vi "Print File.vi"(8 "error in (no error)":errorcluster, 9 "#Copies (1)":i16=1, 10 "Printer Name (default)":string, 11 "File Path":path) -> (0 "error out":errorcluster, 3 "ERROR":bool)   [LabVIEW 2017]
doc: "Prints the document located at the <b>File Path</b> location.\n\nThis VI uses the Windows PrintDocument .NET by creating an instance of the PrintDocument class, setting properties such as the DocumentName and PrinterSettings (PrinterName, number of Copies), and calling the Print method to start the printing process."
uses:
  user32.dll
  shell32.dll
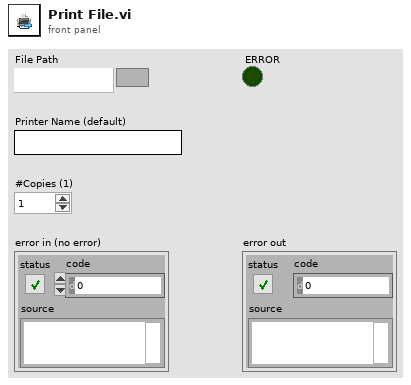
[diagram p1: front panel]
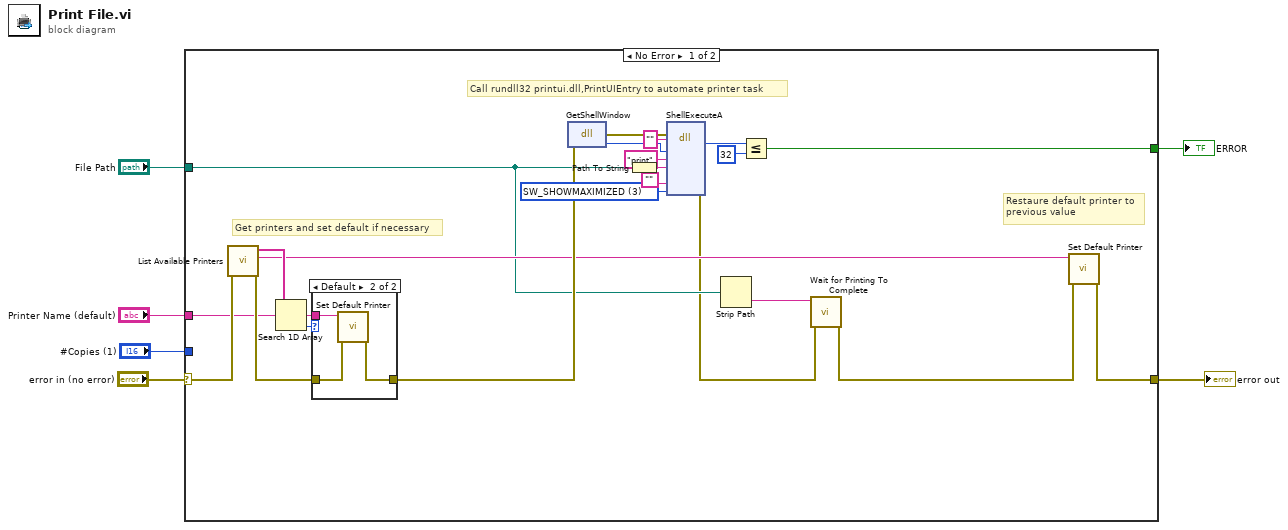
[diagram p0: block diagram]
diagram:
  n1 = case shown="No Error" "error in (no error)" {
    selector: "error in (no error)" -> [w26 w33]
    tunnel: "Printer Name (default)" -> [w12 _]
    tunnel: "File Path" -> [w10 _]
    tunnel: [w19 w33] -> w3
    tunnel: "#Copies (1)" -> [_ _]
    tunnel: [w13 _] -> w1
    frame No Error {
      w16 = u16 3 items=["SW_HIDE", "SW_NORMAL", "SW_SHOWMINIMIZED", "SW_SHOWMAXIMIZED", "SW_SHOWNOACTIVATE", "SW_SHOW", "SW_MINIMIZE", "SW_SHOWMINNOACTIVE", "SW_SHOWNA", "SW_RESTORE", "SW_SHOWDEFAULT", "SW_FORCEMINIMIZE"] ("Flag")
      # "Call rundll32 printui.dll,PrintUIEntry to automate printer task"
      # "Get printers and set default if necessary"
      # "Restaure default printer to\nprevious value"
      n2 = call "List Available Printers.vi"("error in (no error)"=w26) -> ("error out"=w27:errorcluster, "Default Printer"=w11:string, "Available Printers"=w28:string[])  [unwired: 8 in]
      n3 = Search 1D Array(1D array=w28, element=w12) -> (index of element=w14:i32)  [unwired: 1 in]
      n4 = case shown="Default" w14 {
        tunnel: w12 -> [_ w30]
        tunnel: w27 -> [w29 w32]
        tunnel: [w29 w31] -> w20
        frame -1 {
        }
        frame Default {
          n5 = call "Set Default Printer.vi"("error in (no error)"=w32, "Printer Name"=w30) -> ("error out"=w31:errorcluster)  [unwired: 9 in]
        }
      }
      n6 = dll-call lib="user32.dll" fn="GetShellWindow" label="user32.dll -> GetShellWindow"(error in=w20) -> (error out=w25:errorcluster, w24:u32)  [unwired: 2 in, 1 out]
      n7 = Path To String(path=w10) -> (string=w22:string)
      n8 = dll-call lib="shell32.dll" fn="ShellExecuteA" label="shell32.dll ->ShellExecuteA"(error in=w25, "hwnd"=w24, "lpOperation"="print", "lpFile"=w22, "lpParameters"="", "lpDirectory"="" ("lpParameters"), "nShowCmd"=w16) -> (error out=w9:errorcluster, "return type"=w17:i32)  [unwired: 5 in, 4 out]
      n9 = Strip Path(path=w10) -> (name=w7:string)  [unwired: 1 out]
      n10 = Less Or Equal?(x=w17, y=32) -> (x <= y?=w13:bool)
      n11 = call "Wait for Printing To Complete.vi"("error in (no error)"=w9, "File Name"=w7) -> ("error out"=w8:errorcluster)  [unwired: 9 in]
      n12 = call "Set Default Printer.vi"("error in (no error)"=w8, "Printer Name"=w11) -> ("error out"=w19:errorcluster)  [unwired: 9 in]
    }
    frame Error {
    }
  }
  "error out" <- w3
  "ERROR" <- w1
